vi "Get Name.vi"(8 "error in":errorcluster, 11 "Demo in":refnum<class "Demo.lvclass">) -> (0 "error out":errorcluster, 2 "Name":string, 3 "Demo out":refnum<class "Demo.lvclass">)   [LabVIEW 2020, in "Demo.lvclass"]
uses:
  Demo.lvclass
  Demo.lvclass/Demo.ctl
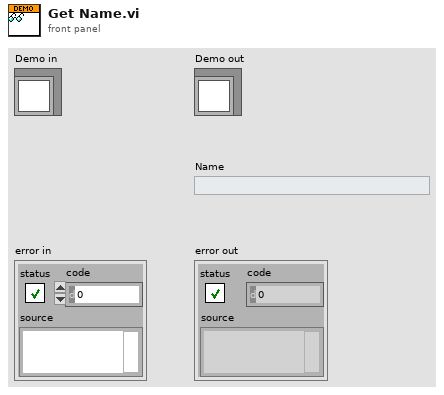
[diagram p1: front panel]
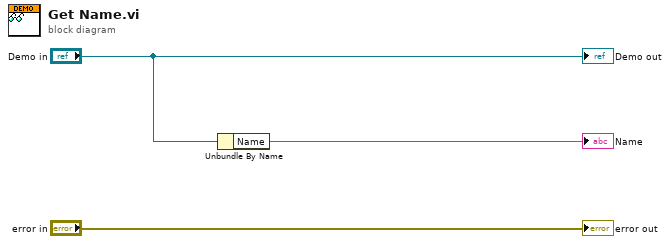
[diagram p0: block diagram]
diagram:
  n1 = Unbundle By Name("Demo in") -> ("Name"=→"Name":string)
  "error out" <- "error in"
  "Demo out" <- "Demo in"
